vi "TracepointLowRateFired.vi"(8 "error in (no error)":errorcluster, 9 "new data":T1, 10 "new block number":u32, 11 "Qbus":refnum<class "Qbus.lvclass">) -> (0 "error out":errorcluster)   [LabVIEW 2017, in "DataAccumulator.lvlib"]
uses:
  <vilib>/addons/InsightCM/Devices/Shared/Common/DataAccumulator/DataAccumulator.lvlib
  <vilib>/addons/Qbus/Qbus.lvclass
  <vilib>/addons/InsightCM/Devices/Shared/Common/DataFlow/controls/Data.ctl
  <vilib>/addons/InsightCM/Utilities/DataAccessors/controls/wfmSGL_DVR.ctl
  <vilib>/addons/PointValueMap/controls/PointMap.ctl
  <vilib>/addons/InsightCM/Devices/Shared/Common/DataFlow/controls/Type.ctl
  <vilib>/addons/TraceLogger/TraceLogger.lvlib
  <vilib>/addons/PointValueMap/PointValueMap.lvlib
  <vilib>/addons/InsightCM/Devices/Shared/Common/DataFlow/DataFlow.lvlib
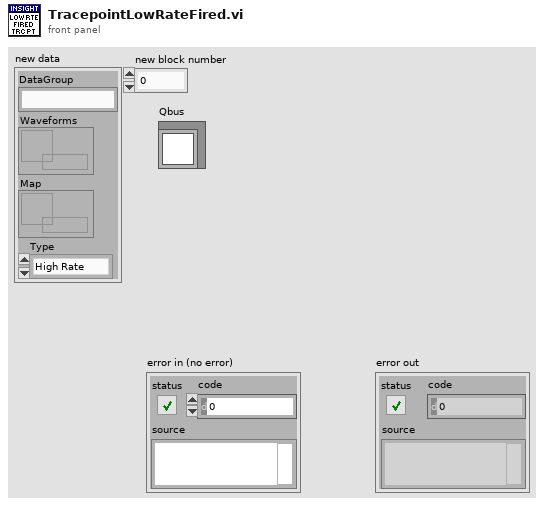
[diagram p1: front panel]
types:
  T1 = typedef "DataFlow.lvlib/Data.ctl" = cluster{"DataGroup":string, "Waveforms":T2, "Map":T3, "Type":T4}
  T2 = typedef "wfmSGL_DVR.ctl" = refnum<data-value>
  T3 = typedef "PointValueMap.lvlib/PointMap.ctl" = refnum<data-value>
  T4 = typedef "DataFlow.lvlib/Type.ctl" = enum16{"High Rate", "Low Rate", "Burst Mode"}
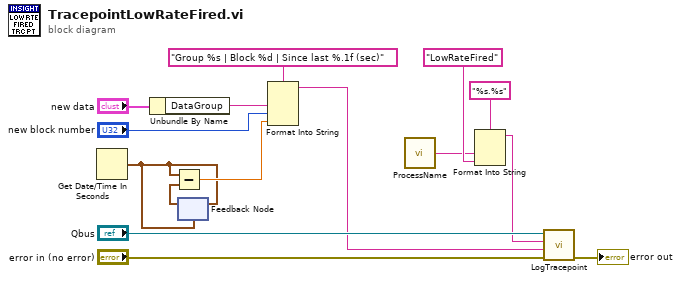
[diagram p0: block diagram]
diagram:
  n1 = Get Date/Time In Seconds() -> (seconds since 1Jan1904=w1:timestamp)
  n2 = Unbundle By Name("new data") -> ("DataGroup"=w5:string)
  n3 = feedback #1(w1) -> (w4:timestamp)
  n4 = Subtract(x=w1, y=w4) -> (x-y=w3:dbl)
  n5 = feedback-in #1(w1) -> ()
  n6 = Format Into String(format string="Group %s | Block %d | Since last %.1f (sec)", w5, "new block number", w3) -> (resulting string=w7:string)  [unwired: 2 in, 1 out]
  n7 = call <vilib>:"ProcessName.vi"() -> ("process name"=w11:string)  [unwired: 5 in]
  n8 = Format Into String(format string="%s.%s", w11, "LowRateFired" ("tracepoint")) -> (resulting string=w12:string)  [unwired: 2 in, 1 out]
  n9 = call <vilib>:"LogTracepoint.vi"("error in (no error)"="error in (no error)", "log string"=w7, "tracepoint"=w12, "qbus in"="Qbus") -> ("error out"=→"error out":errorcluster)  [unwired: 6 in, 1 out]
